vi "To Well Known Type.vi"(1 "message name":string) -> (0 "well known type":T1)   [LabVIEW 2019, in "grpc-lvsupport.lvlib"]
uses:
  grpc-lvsupport.lvlib
  Well Known Types.ctl
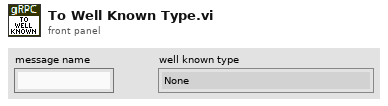
[diagram p1: front panel]
types:
  T1 = typedef "grpc-lvsupport.lvlib/Well Known Types.ctl" = enum32{"None", "Double2DArray", "String2DArray"}
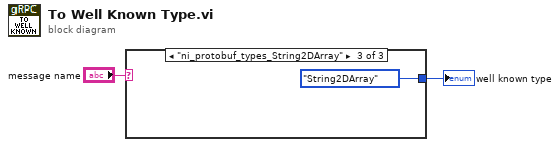
[diagram p0: block diagram]
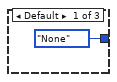
[diagram p2: hidden frame]
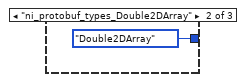
[diagram p3: hidden frame]
diagram:
  n1 = case shown="\"ni_protobuf_types_String2DArray\"" "message name" {
    tunnel: [Well_Known_Types."None" ("Well Known Types") Well_Known_Types."Double2DArray" ("Well Known Types") Well_Known_Types."String2DArray" ("Well Known Types")] -> w1
    frame Default {
    }
    frame "ni_protobuf_types_Double2DArray" {
    }
    frame "ni_protobuf_types_String2DArray" {
    }
  }
  "well known type" <- w1
